vi "Symphony Operate.vi"() -> ()   [LabVIEW 2019]
uses:
  <userlib>/JY Symphony/NoiseCorr.ctl
  <userlib>/JY Symphony/AcqParState.ctl
  <userlib>/JY Symphony/SetAcqParMessage.ctl
panel:
  in  "Noise Corr":T1 caption="Noise Substraction"
  in  "SetArea":bool
  in  "Y Start":i32=255 min=1 max=255 step=1
  in  "X End":i32=1024 min=1 max=1024 step=1
  in  "Y End":i32=256 min=1 max=256 step=1
  in  "X Start":i32=1023 min=1 max=1023 step=1
  out "RemCom":bool
  in  "Server Running":bool
  out "TempReq":bool
  in  "Image mode":bool
  in  "T_Acq_Int":u32=1000 caption="T_Acq_Interval (ms)"
  out "T_AcqTime":u32
  out "Aquiring":bool
  out "Current Temp":dbl
  in  "ReadTemp":bool
  in  "Continuous Acq.":bool
  in  "AcquireImage":bool
  in  "Y Bins":i32=1 min=1 max=256 step=1
  out "ServerConn":refnum<k13>
  in  "Launch server":bool
  out "ClientConn":refnum<k13>
  out "Datas":i32[][][](array[numeric])
  out "Acq Time(ms)":u32
  in  "Accumulations":u16=1 min=1 step=1
  in  "Shutter Enable":bool=TRUE
  in  "Areas":i32[][](array[numeric])=[[1], [1], [1], [1024], [256], [1], [1]]
  in  "Int_time(ms)":u16=10 caption="Integration time(ms)"
  out "Initialized":bool
  in  "ADC":u16(ring) caption="Device Name" items=["ADC1:  20 kHz Tab 1", "ADC1:  50 kHz Tab 2"]
  in  "Gain":u16(ring) caption="Device Name" items=["Gain  0.6(x)"=10, "Gain  1.0(x)"=11, "Gain  2.0(x)"=12, "Gain  4.0(x)"=13, "Gain  6.7(x)"=8, "Gain 13.3(x)"=2]
  out "Name":string="ccd de test"
  out "FirmwareVersion":string="V1.89  CCD_3000"
  out "activeXPixels":i32=1024
  out "activeYPixels":i32=256
  in  "Uniques ID":u16(ring) items=["CCD100"]
  in  "Camera Name":u16(ring) items=["Symphony"]
  in  "Stop":bool
  out "error out":errorcluster
  in  "Init":bool
  in  "error in (no error)":errorcluster
  in  "Tab Control":enum32{"Spectre", "Image"}(tab)
  out "Delta":i32
  out "Max X Position":i32[](array[numeric])
  out "Spectral Graph":i32[][](graph)
  out "Max Intensity":i32[](array[numeric])
  out "Image Graph":i32[][](graph)
  # "Area#"
  # "X Origin"
  # "Y Origin"
  # "X Size"
  # "Y Size"
  # "X Bin"
  # "Y Bin"
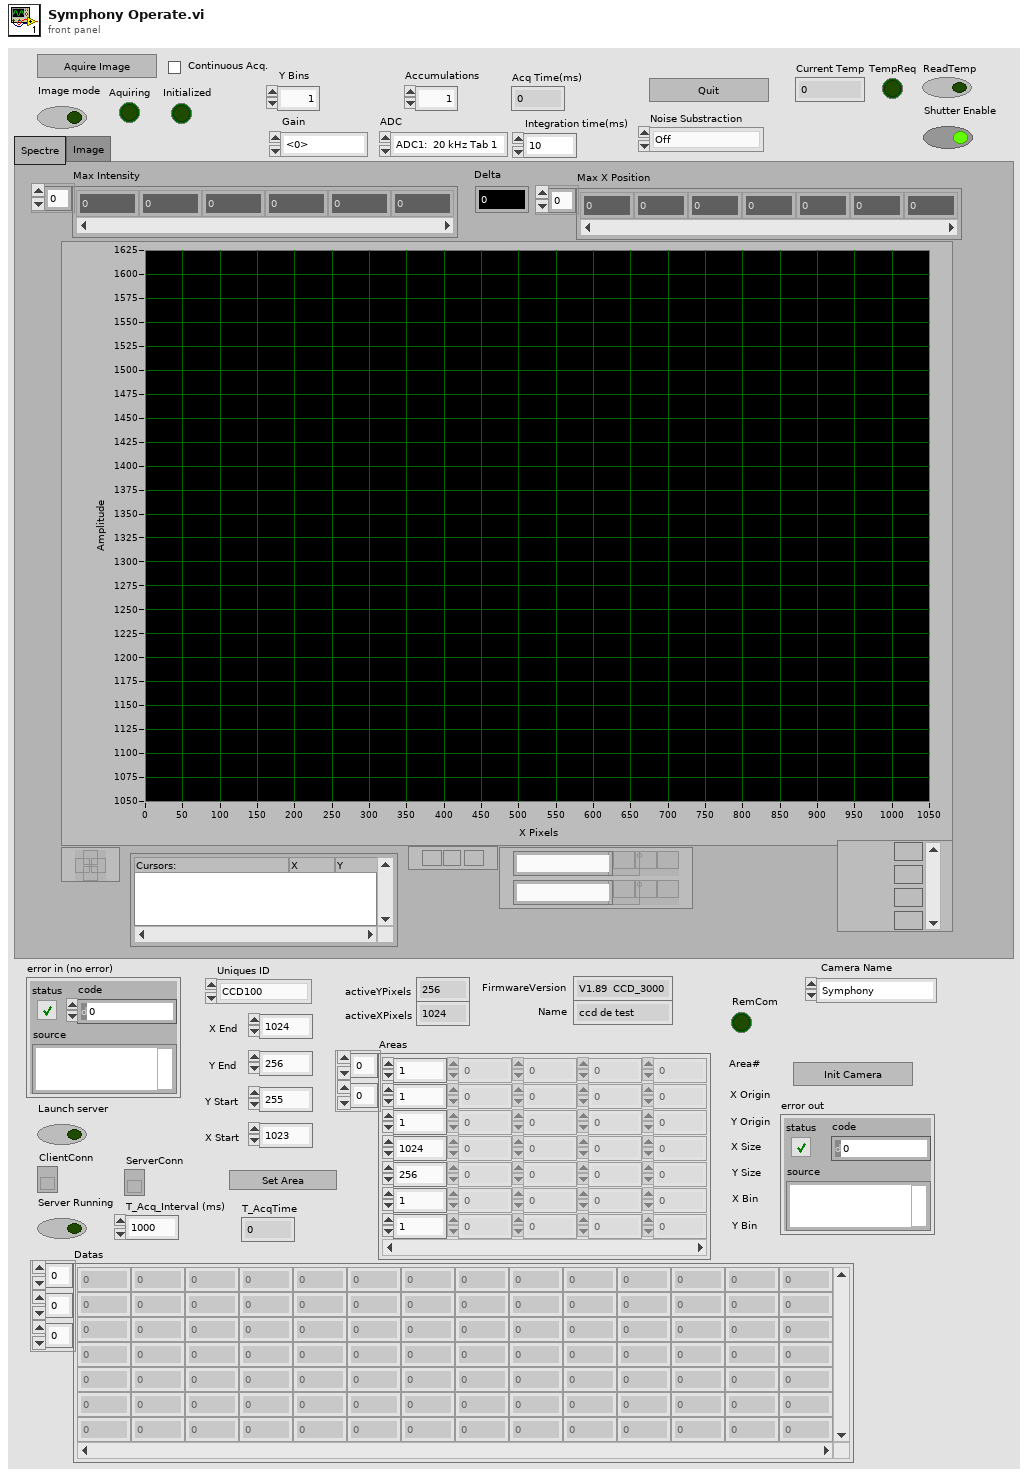
[diagram p1: front panel]
types:
  T1 = typedef "NoiseCorr.ctl" = enum16{"Off", "One For All Acq", "One For Every Acq"}
  T2 = cluster{"Message":string, "Data":variant, "Code":i32}
  T3 = enum16{"Read", "Write", "ReadWrite", "BufferedRead", "BufferedReadWrite"}
  T4 = typedef "AcqParState.ctl" = enum16{"All", "ADC", "Gain", "AcqType", "IntegTime", "Areas", "Error"}
  T5 = typedef "SetAcqParMessage.ctl" = cluster{"ADC":u16, "Gain":u16, "Int_time(ms)":u16, "Areas":i32[][], "Accumulation":u16}
  T6 = cluster{"Description":string, "GetNextADC":u16}[]
  T7 = typedef "LVStringsAndValuesArrayTypeDef_U16.ctl" = cluster{"String":string, "Value":u16}[]
  T8 = cluster{"StringsAndValues[]":T7, "Value":u16, "StringsAndValues[]":T7, "Value":u16, "Int_time(ms)":u16, "Areas":i32[][], "Current Temp":dbl, "Image mode":bool, "Shutter Enable":bool, "Accumulations":u16, u16}
  T9 = cluster{"Datas":i32[][][], "Current Temperature":dbl, "Image mode":bool}
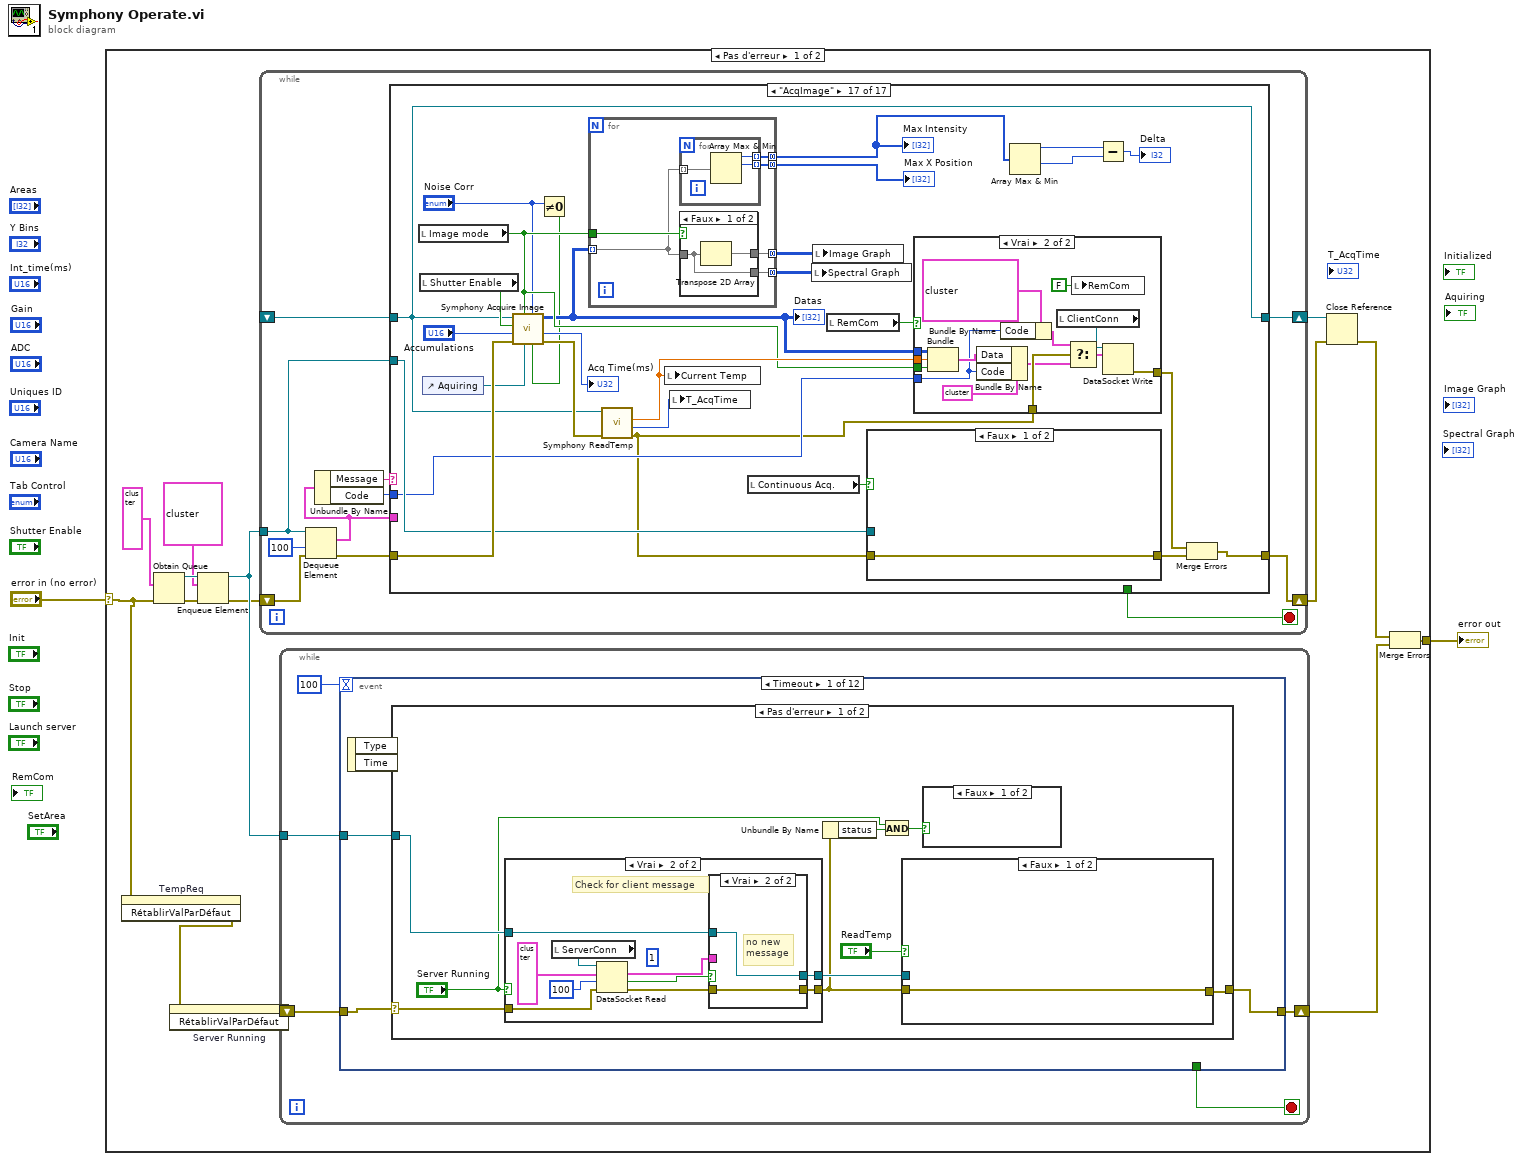
[diagram p0: block diagram]
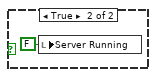
[diagram p2: hidden frame]
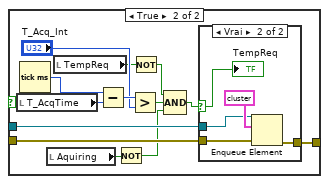
[diagram p3: hidden frame]
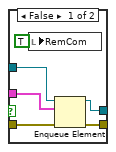
[diagram p6: hidden frame]
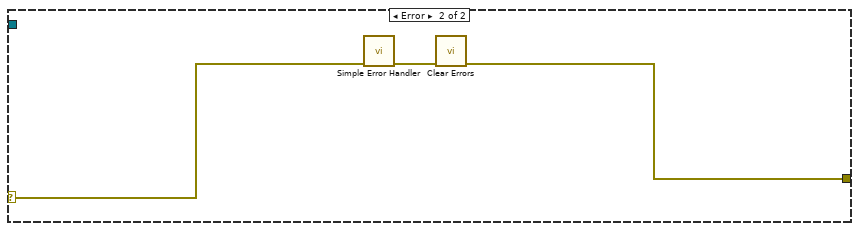
[diagram p7: hidden frame]
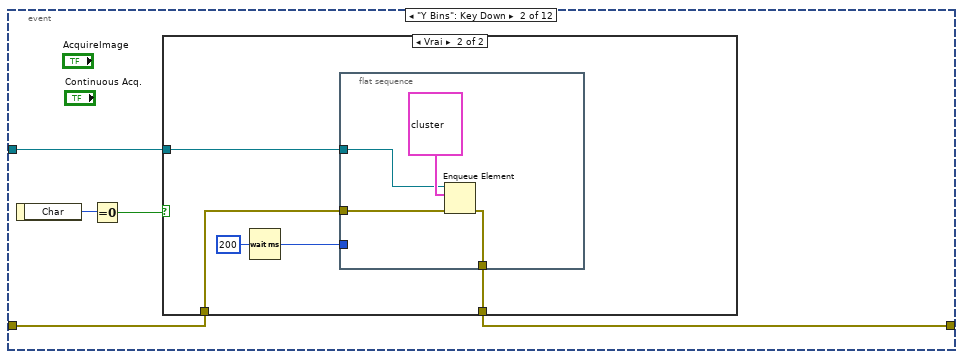
[diagram p8: hidden frame]
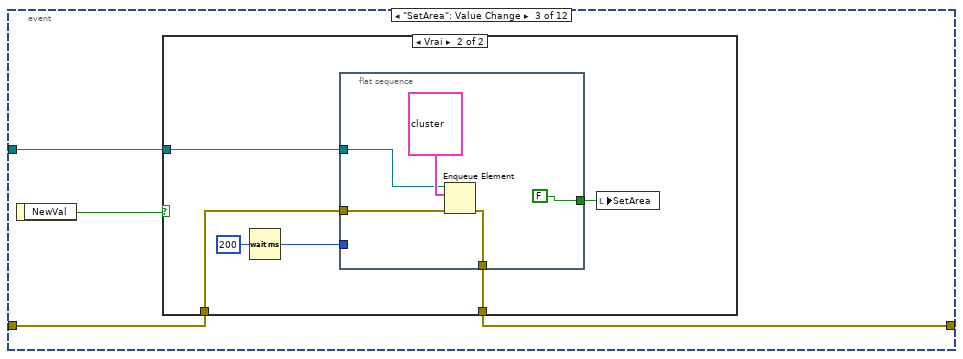
[diagram p10: hidden frame]
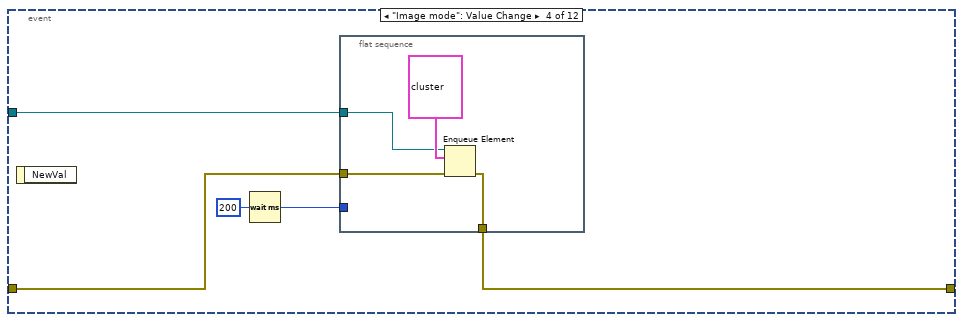
[diagram p12: hidden frame]
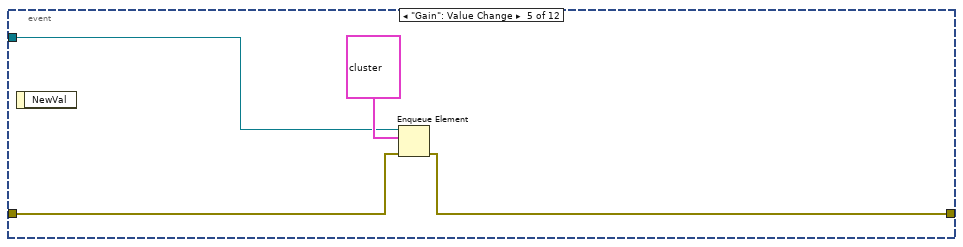
[diagram p13: hidden frame]
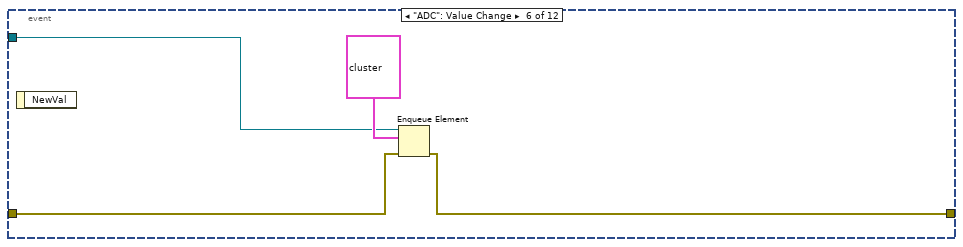
[diagram p14: hidden frame]
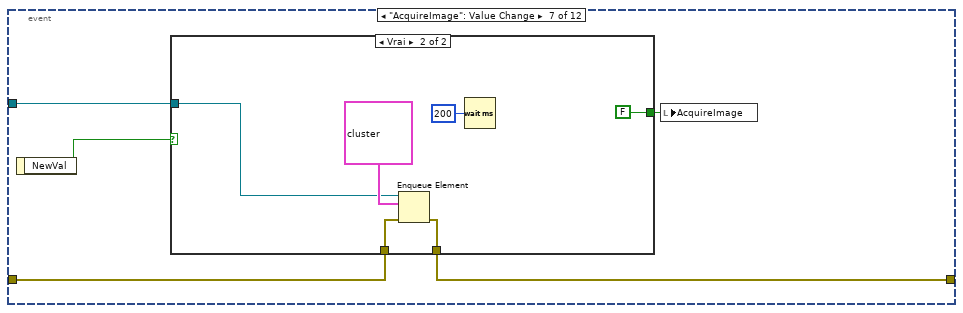
[diagram p15: hidden frame]
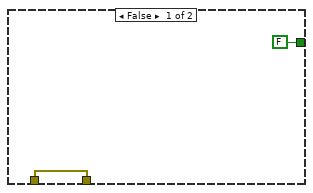
[diagram p16: hidden frame]
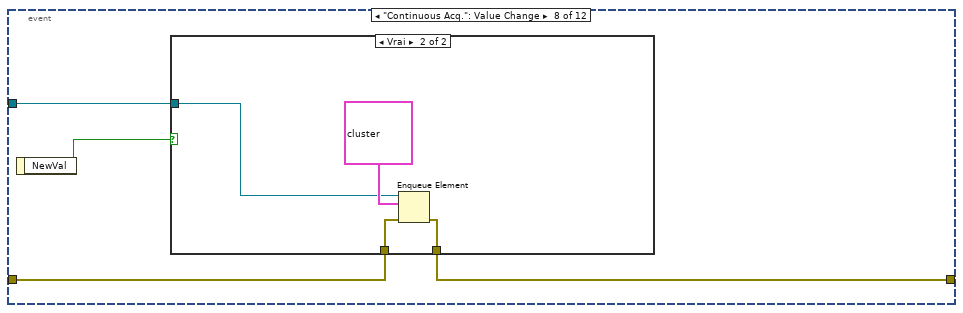
[diagram p17: hidden frame]
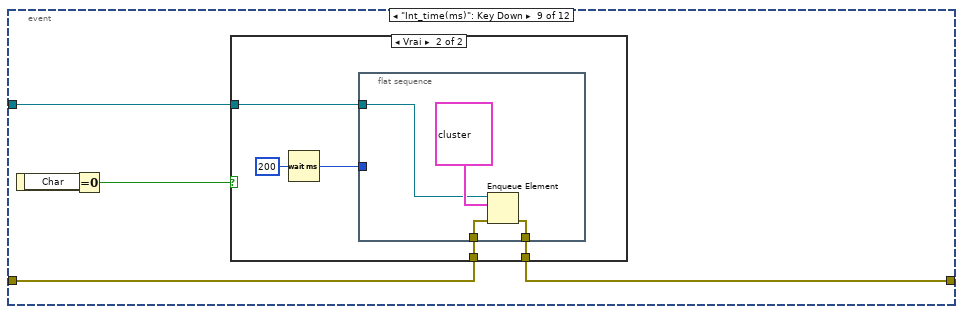
[diagram p19: hidden frame]
diagram:
  n1 = case shown="Pas d'erreur" "error in (no error)" {
    selector: "error in (no error)" -> [w4 w721]
    tunnel: [w14 w721] -> w1
    frame No Error {
      n2 = invoke on="TempReq" class="Bool (strict)" method="RétablirValParDéfaut"(error in=w4) -> (error out=w3:errorcluster)  [unwired: 2 in, 2 out]
      n3 = Obtain Queue(element data type=T2 {"Message"="", "Data"=variant, "Code"=0} ("element"), error in (no error)=w4) -> (queue out=w15:refnum<queue>, error out=w16:errorcluster)  [unwired: 3 in, 1 out]
      n4 = invoke on="Server Running" class="Bool (strict)" method="RétablirValParDéfaut"(error in=w3) -> (error out=w6:errorcluster)  [unwired: 2 in, 2 out]
      n5 = Enqueue Element(queue=w15, element=cluster{"Message":string, "Data":variant, i32} {"Message"="Init Prog", "Data"=variant, 0} ("ClassQueue"), error in (no error)=w16) -> (queue out=w13:refnum<queue>, error out=w5:errorcluster)  [unwired: 1 in, 1 out]
      n6 = while {
        shift-right: [w206] -> w8
        shift-left: w5 -> [w207]
        tunnel: w13 -> [w198]
        shift-right: [w202] -> w7
        shift-left: _ -> [w201]
        stop <- w203 stop-if-true
        n7 = Dequeue Element(queue=w198, timeout in ms (-1)=100, error in (no error)=w207) -> (element=w199:T2, error out=w205:errorcluster)  [unwired: 2 out]
        n8 = Unbundle By Name(w199) -> ("Message"=w204:string, "Code"=w197:i32)
        n9 = case shown="\"AcqImage\"" w204 {
          tunnel: [w208 w222 w245 w278 w319 w323 w351 w376 w423 w452 w487 w522 w556 w583 w608 w642 w664] -> w206
          tunnel: w205 -> [w209 w225 w232 w282 w314 w344 w350 w381 w428 w451 w486 w521 w555 w582 w611 w652 w682]
          tunnel: [TRUE FALSE FALSE _ _ _ _ _ _ _ _ _ _ _ _ _ _] -> w203
          tunnel: [w211 w223 w251 w292 w318 w321 w349 w375 w422 w453 w488 w523 w557 w584 w609 w641 w673] -> w202
          tunnel: w201 -> [w211 w223 w251 _ w313 w343 w349 w380 w427 w454 w489 w524 w558 w585 w610 w641 w673]
          tunnel: w199 -> [_ _ _ _ _ _ _ w378 w425 w450 w485 w520 w554 w581 _ w654 _]
          tunnel: w198 -> [_ _ w248 w276 _ _ _ _ _ _ _ _ _ _ _ w651 w676]
          tunnel: w197 -> [_ _ _ _ _ _ w348 w377 w424 w449 w484 w519 w553 w580 w606 _ w662]
          frame "Stop" {
            n10 = local read "Launch server"() -> (w210:bool)
            n11 = case shown="Vrai" w210 {
              tunnel: w209 -> [w213 w219]
              tunnel: [w213 w215] -> w208
              frame False {
              }
              frame True {
                n12 = local read "ServerConn"() -> (w218:refnum<k13>)
                n13 = local read "ClientConn"() -> (w220:refnum<k13>)
                n14 = DataSocket Close(8:w219, 11:w218) -> (0:w216:errorcluster)  [unwired: 1 in, 1 out]
                n15 = DataSocket Close(8:w219, 11:w220) -> (0:w217:errorcluster)  [unwired: 1 in, 1 out]
                n16 = local write "Server Running"(FALSE ("Server Running")) -> ()
                n17 = Merge Errors(w216, w217) -> (w215:errorcluster)
              }
            }
          }
          frame "Timeout", Default {
            n18 = call <vilib>:"General Error Handler.vi"("error in (no error)"=w225) -> ("error out"=w221:errorcluster)  [unwired: 10 in, 4 out]
            n19 = local write "error out"(w221) -> ()
            n20 = call <vilib>:"Clear Errors.vi"("error in (no error)"=w221) -> ("error out"=w222:errorcluster)  [unwired: 5 in, 1 out]
          }
          frame "Init Prog" {
            n21 = invoke on="Initialized" class="Bool (strict)" method="RétablirValParDéfaut"(error in=w232) -> (error out=w242:errorcluster)  [unwired: 2 in, 2 out]
            n22 = call <userlib>:"Symphony Read Det Uniq_ID.vi"("error in (no error)"=w232) -> ("error out"=w252:errorcluster, "Name"=w253:string[], "UniqueID"=w249:string[])  [unwired: 6 in, 2 out]
            n23 = call <userlib>:"Symphony GetProgPar.vi"("Param"=enum16{"InitVal", "Tous"}."InitVal", "error in"=w232) -> ("InitOnStart"=w233:bool, "Launch server"=w234:bool, "error out"=w229:errorcluster)  [unwired: 3 in, 8 out]
            n24 = Reverse 1D Array(array=u32[] [16711680, 16773120, 2359040, 131327, 3080307] ("Sous-tableau")) -> (reversed array=w243:u32[])
            n25 = property on="Camera Name" class="MDér (strict)"(error in=w252, "Strings []"=w253) -> (error out=w250:errorcluster)  [unwired: 1 in, 1 out]
            n26 = invoke on="Y Bins" class="DigNum (strict)" method="RétablirValParDéfaut"(error in=w242) -> (error out=w241:errorcluster)  [unwired: 2 in, 2 out]
            n27 = local write "Launch server"(w234) -> ()
            n28 = property on="Uniques ID" class="MDér (strict)"(error in=w250, "Strings []"=w249) -> (error out=w231:errorcluster)  [unwired: 1 in, 1 out]
            n29 = for {
              tunnel: cluster{dbl, u32}[] [{0.0, 0}, {10923.0, 0}, {21845.0, 0}, {32768.0, 0}, {43691.0, 0}, {54613.0, 0}] ("Z Scale.Marker Values[]") -> [w257] mode=indexing
              tunnel: w243 -> [w256] mode=indexing
              tunnel: [w255] -> w238 mode=indexing
              n30 = Bundle(cluster=w257, w256) -> (w255:cluster{dbl, u32})  [unwired: 1 in]
            }
            n31 = invoke on="Accumulations" class="DigNum (strict)" method="RétablirValParDéfaut"(error in=w241) -> (error out=w240:errorcluster)  [unwired: 2 in, 2 out]
            n32 = Merge Errors(w231, w229) -> (w230:errorcluster)
            n33 = invoke on="Areas" class="Arr (strict)" method="RétablirValParDéfaut"(error in=w240) -> (error out=w236:errorcluster)  [unwired: 2 in, 2 out]
            n34 = case shown="Vrai" w234 {
              tunnel: [w263 w266] -> w246
              tunnel: w230 -> [w263 w269]
              frame False {
              }
              frame True {
                n35 = DataSocket Open(8:w269, 10:T3."Write" ("mode"), 11:"dstp://localhost/SympClient" ("URL")) -> (0:w271:errorcluster, 3:→"ClientConn":refnum<k13>)  [unwired: 1 in]
                n36 = DataSocket Open(8:w271, 10:T3."Read" ("mode"), 11:"dstp://localhost/SympServer" ("URL")) -> (0:w266:errorcluster, 3:→"ServerConn":refnum<k13>)  [unwired: 1 in]
                n37 = Unbundle By Name(w266) -> ("status"=w265:bool)
                n38 = Not(x=w265) -> (.not. x?=w264:bool)
                n39 = local write "Server Running"(w264) -> ()
              }
            }
            n40 = property on="Image Graph" class="GraphInt (strict)"(error in=w232, "ZScale.MarkerVals[]"=w238) -> (error out=w239:errorcluster)  [unwired: 1 in, 1 out]
            n41 = invoke on="Image mode" class="Bool (strict)" method="RétablirValParDéfaut"(error in=w236) -> (error out=w235:errorcluster)  [unwired: 2 in, 2 out]
            n42 = case shown="Vrai" w233 {
              tunnel: w248 -> [_ w261]
              tunnel: w230 -> [w258 w260]
              tunnel: [w258 w259] -> w247
              frame False {
              }
              frame True {
                n43 = Enqueue Element(queue=w261, element=cluster{"Message":string, "Data":variant, i32} {"Message"="InitCam", "Data"=variant, 0} ("ClassQueue"), error in (no error)=w260) -> (error out=w259:errorcluster)  [unwired: 1 in, 2 out]
              }
            }
            n44 = invoke on="RemCom" class="Bool (strict)" method="RétablirValParDéfaut"(error in=w235) -> (error out=w227:errorcluster)  [unwired: 2 in, 2 out]
            n45 = invoke on="Noise Corr" class="Enum (strict)" method="RétablirValParDéfaut"(error in=w227) -> (error out=w226:errorcluster)  [unwired: 2 in, 2 out]
            n46 = Merge Errors(w226, w246, w247, w239) -> (w245:errorcluster)
          }
          frame "InitCam" {
            n47 = call <vilib>:"Set Busy.vi"("error in (no error)"=w282) -> ("error out"=w281:errorcluster)  [unwired: 9 in, 1 out]
            n48 = local read "Camera Name"() -> (w300:u16)
            n49 = property on="Uniques ID" class="MDér (strict)"(error in=w281) -> (error out=w297:errorcluster, "Strings []"=w301:string[])  [unwired: 1 in, 1 out]
            n50 = To Long Integer(number=w300) -> (32bit integer=w299:i32)
            n51 = Index Array(array=w301, index=w299) -> (element=w298:string)
            n52 = call <userlib>:"Symphony Init.vi"("error In"=w297, "Unique id:"=w298) -> ("error out"=w293:errorcluster, "activeYPixels"=→"activeYPixels":i32, "activeXPixels"=→"activeXPixels":i32, "JYCCDLib.IJYCCDReqd"=w294:refnum<k7>, "Name"=→"Name":string, "FirmwareVersion"=→"FirmwareVersion":string)  [unwired: 3 in]
            n53 = call <userlib>:"Symphony Init ADC & Gain.vi"("error in (no error)"=w293, "JYCCDLib.IJYCCDReqd"=w294) -> ("error out"=w291:errorcluster, "ADC Values"=w289:T6, "Gain Values"=w284:T6, "JYCCDLib.IJYCCDReqd Out"=w292:refnum<k7>, "CurrentADC"=w287:i32, "CurrentGain"=w285:i32)  [unwired: 4 in]
            n54 = To Unsigned Word Integer(number=w285) -> (unsigned 16bit integer=w286:u16)
            n55 = To Unsigned Word Integer(number=w287) -> (unsigned 16bit integer=w283:u16)
            n56 = property on="ADC" class="MDér (strict)"(error in=w291, "StringsAndValues[]"=w289, "Value"=w283) -> (error out=w288:errorcluster)  [unwired: 1 in, 1 out]
            n57 = property on="Gain" class="MDér (strict)"(error in=w291, "StringsAndValues[]"=w284, "Value"=w286) -> (error out=w290:errorcluster)  [unwired: 1 in, 1 out]
            n58 = Merge Errors(w290, w288) -> (w277:errorcluster)
            n59 = case shown="Pas d'erreur" w277 {
              selector: w277 -> [w306 w308]
              tunnel: w276 -> [w305 _]
              tunnel: [w304 w308] -> w275
              frame No Error {
                n60 = Enqueue Element(queue=w305, element=T2 {"Message"="InitSetupAll", "Data"=variant, "Code"=1}, error in (no error)=w306) -> (error out=w304:errorcluster)  [unwired: 1 in, 2 out]
              }
              frame Error {
              }
            }
            n61 = call <vilib>:"Clear Errors.vi"("error in (no error)"=w277) -> ("error out"=w280:errorcluster)  [unwired: 5 in, 1 out]
            n62 = call <vilib>:"Unset Busy.vi"("error in (no error)"=w280) -> ("error out"=w279:errorcluster)  [unwired: 10 in]
            n63 = Merge Errors(w275, w279) -> (w278:errorcluster)
          }
          frame "AcqSetupAll" {
            (unwired) 0 ("Code")
            n64 = local read "Int_time(ms)"() -> (w312:u16)
            n65 = local read "Areas"() -> (w309:i32[][])
            n66 = local read "ADC"() -> (w311:u16)
            n67 = local read "Gain"() -> (w310:u16)
            n68 = To Long Integer(number=w311) -> (32bit integer=w316:i32)
            n69 = To Long Integer(number=w310) -> (32bit integer=w317:i32)
            n70 = call <userlib>:"Symphony Setup V2.vi"("areas :"=w309, "Function"=AcqParState."All", "Int_time(ms)"=w312, "error in (no error)"=w314, "Gain"=w317, "Select ADC"=w316, "JYCCDLib.IJYCCDReqd"=w313) -> ("error out"=w319:errorcluster, "JYCCDLib.IJYCCDReqdOut"=w318:refnum<k7>)  [unwired: 2 in, 1 out]
          }
          frame "InitSetupAll" {
            w326 = u16 0 items=["° Celsius", "Kelvin", "° Farenheit"] ("units")
            w338 = 256 ("Y Start")
            w340 = 1 ("Y Start")
            n71 = call <userlib>:"Symphony GetProgPar.vi"("Param"=enum16{"InitVal", "Tous"}."Tous", "error in"=w344) -> ("Y Bins"=w335:i32, "X Start"=w337:i32, "X End"=w339:i32, "ImageMode"=w336:bool, "Shutter Enable"=w330:bool, "ADC"=w332:u16, "Gain"=w333:u16, "Int_time(ms)"=w329:i16, "error out"=w342:errorcluster)  [unwired: 3 in, 2 out]
            n72 = local write "Shutter Enable"(w330) -> ()
            n73 = local write "Int_time(ms)"(w329) -> ()
            n74 = local write "Gain"(w333) -> ()
            n75 = local write "ADC"(w332) -> ()
            n76 = local write "Image mode"(w336) -> ()
            n77 = local write "Y Bins"(w335) -> ()
            n78 = local write "X Start"(w337) -> ()
            n79 = local write "X End"(w339) -> ()
            n80 = call <userlib>:"Symphony Format Area.vi"("Y Start"=w340, "Y End"=w338, "ImageMode"=w336, "error in (no error)"=w342, "X Start"=w337, "X End"=w339, "numAreas"=w335) -> ("error out"=w341:errorcluster, "areas :"=w334:i32[][])  [unwired: 1 in, 1 out]
            n81 = local write "Y End"(w338) -> ()
            n82 = local write "Areas"(w334) -> ()
            n83 = local write "Y Start"(w340) -> ()
            n84 = To Long Integer(number=w332) -> (32bit integer=w346:i32)
            n85 = To Long Integer(number=w333) -> (32bit integer=w347:i32)
            n86 = call <userlib>:"Symphony Setup V2.vi"("areas :"=w334, "Function"=AcqParState."All", "Int_time(ms)"=w329, "error in (no error)"=w341, "Gain"=w347, "Select ADC"=w346, "JYCCDLib.IJYCCDReqd"=w343) -> ("error out"=w324:errorcluster, "JYCCDLib.IJYCCDReqdOut"=w322:refnum<k7>)  [unwired: 2 in, 1 out]
            n87 = call <userlib>:"Symphony ReadTemp.vi"("error in (no error)"=w324, "units"=w326, "JYCCDLib.IJYCCDReqd"=w322) -> ("error out"=w323:errorcluster, "AcqTime"=w325:u32, "Current Temperature"=w327:dbl, "reference out"=w321:refnum<k7>)  [unwired: 4 in]
            n88 = local write "T_AcqTime"(w325) -> ()
            n89 = local write "Current Temp"(w327) -> ()
            n90 = Unbundle By Name(w323) -> ("status"=w328:bool)
            n91 = Not(x=w328) -> (.not. x?=w320:bool)
            n92 = local write "Initialized"(w320) -> ()
          }
          frame "CheckStatus" {
            n93 = local read "RemCom"() -> (w352:bool)
            n94 = case shown="Vrai" w352 {
              selector: w352 -> [_ w360]
              tunnel: w350 -> [w353 w371]
              tunnel: [w353 w370] -> w351
              tunnel: w348 -> [_ w362]
              frame False {
              }
              frame True {
                n95 = Not(x=w360) -> (.not. x?=w359:bool)
                n96 = property on="ADC" class="MDér (strict)"() -> ("StringsAndValues[]"=w369:T7, "Value"=w368:u16)  [unwired: 2 in, 2 out]
                n97 = property on="Gain" class="MDér (strict)"() -> ("StringsAndValues[]"=w367:T7, "Value"=w366:u16)  [unwired: 2 in, 2 out]
                n98 = local write "RemCom"(w359) -> ()
                n99 = local read "Accumulations"() -> (w356:u16)
                n100 = local read "Image mode"() -> (w358:bool)
                n101 = local read "Int_time(ms)"() -> (w364:u16)
                n102 = local read "Current Temp"() -> (w361:dbl)
                n103 = local read "Shutter Enable"() -> (w357:bool)
                n104 = local read "Noise Corr"() -> (w355:T1)
                n105 = local read "Areas"() -> (w363:i32[][])
                n106 = To Unsigned Word Integer(number=w355) -> (unsigned 16bit integer=w354:u16)
                n107 = Bundle("StringsAndValues[]"=w369, "Value"=w368, "StringsAndValues[]"=w367, "Value"=w366, "Int_time(ms)"=w364, "Areas"=w363, "Current Temp"=w361, "Image mode"=w358, "Shutter Enable"=w357, "Accumulations"=w356, w354) -> (w365:T8)  [unwired: 1 in]
                n108 = local read "ClientConn"() -> (w374:refnum<k13>)
                n109 = Bundle By Name(cluster=T2 {"Message"="Status", "Data"=variant, "Code"=0} ("ClassQueue"), "Data"=w365, "Code"=w362) -> (w372:T2)
                n110 = DataSocket Write(8:w371, 10:w372, 11:w374) -> (0:w370:errorcluster)  [unwired: 1 in, 2 out]
              }
            }
          }
          frame "SetArea" {
            n111 = local read "RemCom"() -> (w379:bool)
            n112 = case shown="Faux" w379 {
              selector: w379 -> [_ w420]
              tunnel: w381 -> [w394 w411]
              tunnel: w380 -> [w393 w416]
              tunnel: [w392 w415] -> w375
              tunnel: w378 -> [_ w413]
              tunnel: w377 -> [_ w409]
              tunnel: [w384 w405] -> w376
              frame False {
                n113 = local read "Y Bins"() -> (w388:i32)
                n114 = call <userlib>:"Symphony Format Area.vi"("Y Start"="Y Start", "Y End"="Y End", "ImageMode"="Image mode", "error in (no error)"=w394, "X Start"="X Start", "X End"="X End", "numAreas"=w388) -> ("error out"=w390:errorcluster, "areas :"=w389:i32[][])  [unwired: 1 in, 1 out]
                n115 = local write "Areas"(w389) -> ()
                n116 = call <userlib>:"Symphony Setup V2.vi"("areas :"=w389, "Function"=AcqParState."Areas", "error in (no error)"=w390, "JYCCDLib.IJYCCDReqd"=w393) -> ("error out"=w384:errorcluster, "JYCCDLib.IJYCCDReqdOut"=w392:refnum<k7>)  [unwired: 5 in, 1 out]
              }
              frame True {
                w407 = T2 {"Message"="CommandError", "Data"=variant, "Code"=0} ("ClassQueue")
                n117 = Not(x=w420) -> (.not. x?=w421:bool)
                n118 = local write "RemCom"(w421) -> ()
                n119 = Unbundle By Name(w413) -> ("Data"=w412:variant)
                n120 = Bundle("Areas"=i32[][] [[1], [1], [1], [1024], [256], [1], [1]], TRUE) -> (w400:cluster{"Areas":i32[][], bool})  [unwired: 1 in]
                n121 = Variant To Data(error in=w411, type=w400, Variant=w412) -> (data=w414:cluster{"Areas":i32[][], bool}, error out=w410:errorcluster)
                n122 = Unbundle(w414) -> ("Areas"=w398:i32[][], w399:bool)
                n123 = Bundle By Name(cluster=w407, "Code"=w409) -> ()  [unwired: 1 out]
                n124 = call <userlib>:"Symphony Setup V2.vi"("areas :"=w398, "Function"=AcqParState."Areas", "error in (no error)"=w410, "JYCCDLib.IJYCCDReqd"=w416) -> ("error out"=w403:errorcluster, "JYCCDLib.IJYCCDReqdOut"=w415:refnum<k7>)  [unwired: 5 in, 1 out]
                n125 = local write "Image mode"(w399) -> ()
                n126 = local write "Areas"(w398) -> ()
                n127 = Array Size(array=w398) -> (size(s)=w397:i32[])
                n128 = Bundle By Name(cluster=T2 {"Message"="Area", "Data"=variant, "Code"=0} ("ClassQueue"), "Code"=w409) -> (w408:T2)
                n129 = Select(t=w407, s=w403, f=w408) -> (s? t:f=w406:T2)
                n130 = local read "ClientConn"() -> (w418:refnum<k13>)
                n131 = Index Array(array=w397, index=1) -> (element=w395:i32)
                n132 = DataSocket Write(10:w406, 11:w418) -> (0:w404:errorcluster)  [unwired: 2 in, 2 out]
                n133 = local write "Y Bins"(w395) -> ()
                n134 = Merge Errors(w404, w403) -> (w405:errorcluster)
              }
            }
          }
          frame "SetShutterEn" {
            n135 = local read "RemCom"() -> (w426:bool)
            n136 = case shown="Vrai" w426 {
              selector: w426 -> [_ w446]
              tunnel: w428 -> [w429 w441]
              tunnel: w427 -> [w430 w433]
              tunnel: [w430 w433] -> w422
              tunnel: w425 -> [_ w443]
              tunnel: w424 -> [_ w440]
              tunnel: [w429 w436] -> w423
              frame False {
              }
              frame True {
                w438 = T2 {"Message"="CommandError", "Data"=variant, "Code"=0} ("ClassQueue")
                n137 = Not(x=w446) -> (.not. x?=w447:bool)
                n138 = local write "RemCom"(w447) -> ()
                n139 = Unbundle By Name(w443) -> ("Data"=w442:variant)
                n140 = Variant To Data(error in=w441, type=TRUE, Variant=w442) -> (data=w431:bool, error out=w434:errorcluster)
                n141 = local write "Shutter Enable"(w431) -> ()
                n142 = Bundle By Name(cluster=w438, "Code"=w440) -> ()  [unwired: 1 out]
                n143 = Bundle By Name(cluster=T2 {"Message"="ShutterEn", "Data"=variant, "Code"=0} ("ClassQueue"), "Code"=w440, "Data"=w431) -> (w439:T2)
                n144 = Select(t=w438, s=w434, f=w439) -> (s? t:f=w437:T2)
                n145 = local read "ClientConn"() -> (w444:refnum<k13>)
                n146 = DataSocket Write(10:w437, 11:w444) -> (0:w435:errorcluster)  [unwired: 2 in, 2 out]
                n147 = Merge Errors(w435, w434) -> (w436:errorcluster)
              }
            }
          }
          frame "SetGain" {
            n148 = local read "RemCom"() -> (w448:bool)
            n149 = case shown="Vrai" w448 {
              selector: w448 -> [_ w462]
              tunnel: w454 -> [w461 w482]
              tunnel: [w460 w481] -> w453
              tunnel: [w458 w470] -> w452
              tunnel: w451 -> [w457 w468]
              tunnel: w450 -> [_ w480]
              tunnel: w449 -> [_ w466]
              frame False {
                n150 = local read "Gain"() -> (w456:u16)
                n151 = To Long Integer(number=w456) -> (32bit integer=w455:i32)
                n152 = call <userlib>:"Symphony Setup V2.vi"("Function"=AcqParState."Gain", "error in (no error)"=w457, "Gain"=w455, "JYCCDLib.IJYCCDReqd"=w461) -> ("error out"=w458:errorcluster, "JYCCDLib.IJYCCDReqdOut"=w460:refnum<k7>)  [unwired: 5 in, 1 out]
              }
              frame True {
                n153 = Not(x=w462) -> (.not. x?=w463:bool)
                n154 = Unbundle By Name(w480) -> ("Data"=w473:variant)
                n155 = local write "RemCom"(w463) -> ()
                n156 = Variant To Data(error in=w468, type=0 ("Gain"), Variant=w473) -> (data=w464:i32, error out=w471:errorcluster)
                n157 = call <userlib>:"Symphony Setup V2.vi"("Function"=AcqParState."Gain", "error in (no error)"=w471, "Gain"=w464, "JYCCDLib.IJYCCDReqd"=w482) -> ("error out"=w469:errorcluster, "JYCCDLib.IJYCCDReqdOut"=w481:refnum<k7>)  [unwired: 5 in, 1 out]
                n158 = Bundle By Name(cluster=T2 {"Message"="Gain", "Data"=variant, "Code"=0} ("ClassQueue"), "Data"=w464, "Code"=w466) -> (w476:T2)
                n159 = local write "Gain"(w464) -> ()
                n160 = Bundle By Name(cluster=T2 {"Message"="CommandError", "Data"=variant, "Code"=0} ("ClassQueue"), "Code"=w466) -> (w465:T2)
                n161 = Select(t=w465, s=w469, f=w476) -> (s? t:f=w477:T2)
                n162 = local read "ClientConn"() -> (w478:refnum<k13>)
                n163 = DataSocket Write(10:w477, 11:w478) -> (0:w474:errorcluster)  [unwired: 2 in, 2 out]
                n164 = Merge Errors(w474, w469) -> (w470:errorcluster)
              }
            }
          }
          frame "SetADC" {
            n165 = local read "RemCom"() -> (w483:bool)
            n166 = case shown="Vrai" w483 {
              selector: w483 -> [_ w497]
              tunnel: w489 -> [w496 w517]
              tunnel: [w495 w516] -> w488
              tunnel: [w493 w505] -> w487
              tunnel: w486 -> [w492 w503]
              tunnel: w485 -> [_ w515]
              tunnel: w484 -> [_ w501]
              frame False {
                n167 = local read "ADC"() -> (w491:u16)
                n168 = To Long Integer(number=w491) -> (32bit integer=w490:i32)
                n169 = call <userlib>:"Symphony Setup V2.vi"("Function"=AcqParState."ADC", "error in (no error)"=w492, "Gain"=w490, "JYCCDLib.IJYCCDReqd"=w496) -> ("error out"=w493:errorcluster, "JYCCDLib.IJYCCDReqdOut"=w495:refnum<k7>)  [unwired: 5 in, 1 out]
              }
              frame True {
                n170 = Unbundle By Name(w515) -> ("Data"=w508:variant)
                n171 = Not(x=w497) -> (.not. x?=w498:bool)
                n172 = local write "RemCom"(w498) -> ()
                n173 = Variant To Data(error in=w503, type=0 ("Gain"), Variant=w508) -> (data=w499:i32, error out=w506:errorcluster)
                n174 = call <userlib>:"Symphony Setup V2.vi"("Function"=AcqParState."ADC", "error in (no error)"=w506, "Gain"=w499, "JYCCDLib.IJYCCDReqd"=w517) -> ("error out"=w504:errorcluster, "JYCCDLib.IJYCCDReqdOut"=w516:refnum<k7>)  [unwired: 5 in, 1 out]
                n175 = Bundle By Name(cluster=T2 {"Message"="ADC", "Data"=variant, "Code"=0} ("ClassQueue"), "Data"=w499, "Code"=w501) -> (w511:T2)
                n176 = local write "ADC"(w499) -> ()
                n177 = Bundle By Name(cluster=T2 {"Message"="CommandError", "Data"=variant, "Code"=0} ("ClassQueue"), "Code"=w501) -> (w500:T2)
                n178 = local read "ClientConn"() -> (w513:refnum<k13>)
                n179 = Select(t=w500, s=w504, f=w511) -> (s? t:f=w512:T2)
                n180 = DataSocket Write(10:w512, 11:w513) -> (0:w509:errorcluster)  [unwired: 2 in, 2 out]
                n181 = Merge Errors(w509, w504) -> (w505:errorcluster)
              }
            }
          }
          frame "SetInteg" {
            n182 = local read "RemCom"() -> (w518:bool)
            n183 = case shown="Vrai" w518 {
              selector: w518 -> [_ w531]
              tunnel: w524 -> [w530 w547]
              tunnel: [w529 w546] -> w523
              tunnel: [w527 w540] -> w522
              tunnel: w521 -> [w526 w538]
              tunnel: w520 -> [_ w551]
              tunnel: w519 -> [_ w533]
              frame False {
                n184 = local read "Int_time(ms)"() -> (w525:u16)
                n185 = call <userlib>:"Symphony Setup V2.vi"("Function"=AcqParState."IntegTime", "Int_time(ms)"=w525, "error in (no error)"=w526, "JYCCDLib.IJYCCDReqd"=w530) -> ("error out"=w527:errorcluster, "JYCCDLib.IJYCCDReqdOut"=w529:refnum<k7>)  [unwired: 5 in, 1 out]
              }
              frame True {
                n186 = Not(x=w531) -> (.not. x?=w532:bool)
                n187 = Unbundle By Name(w551) -> ("Data"=w550:variant)
                n188 = local write "RemCom"(w532) -> ()
                n189 = Variant To Data(error in=w538, type=u16 10 ("Int_time(ms)"), Variant=w550) -> (data=w536:u16, error out=w537:errorcluster)
                n190 = call <userlib>:"Symphony Setup V2.vi"("Function"=AcqParState."IntegTime", "Int_time(ms)"=w536, "error in (no error)"=w537, "JYCCDLib.IJYCCDReqd"=w547) -> ("error out"=w541:errorcluster, "JYCCDLib.IJYCCDReqdOut"=w546:refnum<k7>)  [unwired: 5 in, 1 out]
                n191 = Bundle By Name(cluster=T2 {"Message"="Integration", "Data"=variant, "Code"=0} ("ClassQueue"), "Data"=w536, "Code"=w533) -> (w542:T2)
                n192 = Bundle By Name(cluster=T2 {"Message"="CommandError", "Data"=variant, "Code"=0} ("ClassQueue"), "Code"=w533) -> (w534:T2)
                n193 = local read "ClientConn"() -> (w544:refnum<k13>)
                n194 = local write "Int_time(ms)"(w536) -> ()
                n195 = Select(t=w534, s=w541, f=w542) -> (s? t:f=w543:T2)
                n196 = DataSocket Write(10:w543, 11:w544) -> (0:w539:errorcluster)  [unwired: 2 in, 2 out]
                n197 = Merge Errors(w539, w541) -> (w540:errorcluster)
              }
            }
          }
          frame "SetAcc" {
            n198 = local read "RemCom"() -> (w552:bool)
            n199 = case shown="Vrai" w552 {
              selector: w552 -> [_ w564]
              tunnel: w558 -> [w560 w561]
              tunnel: [w560 w561] -> w557
              tunnel: [w559 w571] -> w556
              tunnel: w555 -> [w559 w569]
              tunnel: w554 -> [_ w578]
              tunnel: w553 -> [_ w566]
              frame False {
              }
              frame True {
                n200 = Not(x=w564) -> (.not. x?=w565:bool)
                n201 = Unbundle By Name(w578) -> ("Data"=w577:variant)
                n202 = local write "RemCom"(w565) -> ()
                n203 = Variant To Data(error in=w569, type=u16 10 ("Int_time(ms)"), Variant=w577) -> (data=w563:u16, error out=w562:errorcluster)
                n204 = Bundle By Name(cluster=T2 {"Message"="Accumulation", "Data"=variant, "Code"=0} ("ClassQueue"), "Data"=w563, "Code"=w566) -> (w572:T2)
                n205 = Bundle By Name(cluster=T2 {"Message"="CommandError", "Data"=variant, "Code"=0} ("ClassQueue"), "Code"=w566) -> (w567:T2)
                n206 = local write "Accumulations"(w563) -> ()
                n207 = local read "ClientConn"() -> (w574:refnum<k13>)
                n208 = Select(t=w567, s=w562, f=w572) -> (s? t:f=w573:T2)
                n209 = DataSocket Write(10:w573, 11:w574) -> (0:w570:errorcluster)  [unwired: 2 in, 2 out]
                n210 = Merge Errors(w570, w562) -> (w571:errorcluster)
              }
            }
          }
          frame "SetNoiseMode" {
            n211 = local read "RemCom"() -> (w579:bool)
            n212 = case shown="Vrai" w579 {
              selector: w579 -> [_ w591]
              tunnel: w585 -> [w587 w588]
              tunnel: [w587 w588] -> w584
              tunnel: [w586 w598] -> w583
              tunnel: w582 -> [w586 w596]
              tunnel: w581 -> [_ w605]
              tunnel: w580 -> [_ w593]
              frame False {
              }
              frame True {
                n213 = Not(x=w591) -> (.not. x?=w592:bool)
                n214 = Unbundle By Name(w605) -> ("Data"=w604:variant)
                n215 = local write "RemCom"(w592) -> ()
                n216 = Variant To Data(error in=w596, type=u16 10 ("Int_time(ms)"), Variant=w604) -> (data=w590:u16, error out=w589:errorcluster)
                n217 = Bundle By Name(cluster=T2 {"Message"="NoiseMode", "Data"=variant, "Code"=0} ("ClassQueue"), "Data"=w590, "Code"=w593) -> (w599:T2)
                n218 = Bundle By Name(cluster=T2 {"Message"="CommandError", "Data"=variant, "Code"=0} ("ClassQueue"), "Code"=w593) -> (w594:T2)
                n219 = local read "ClientConn"() -> (w601:refnum<k13>)
                n220 = local write "Noise Corr"(w590) -> ()
                n221 = Select(t=w594, s=w589, f=w599) -> (s? t:f=w600:T2)
                n222 = DataSocket Write(10:w600, 11:w601) -> (0:w597:errorcluster)  [unwired: 2 in, 2 out]
                n223 = Merge Errors(w597, w589) -> (w598:errorcluster)
              }
            }
          }
          frame "AcqTemp" {
            n224 = local read "RemCom"() -> (w607:bool)
            n225 = case shown="Vrai" w607 {
              selector: w607 -> [_ w634]
              tunnel: w611 -> [w619 w639]
              tunnel: w610 -> [w618 w638]
              tunnel: [w617 w622] -> w609
              tunnel: [w613 w623] -> w608
              tunnel: w606 -> [_ w624]
              frame False {
                w616 = u16 0 items=["° Celsius", "Kelvin", "° Farenheit"] ("units")
                n226 = call <userlib>:"Symphony ReadTemp.vi"("error in (no error)"=w619, "units"=w616, "JYCCDLib.IJYCCDReqd"=w618) -> ("error out"=w614:errorcluster, "AcqTime"=w615:u32, "Current Temperature"=w612:dbl, "reference out"=w617:refnum<k7>)  [unwired: 4 in]
                n227 = local write "T_AcqTime"(w615) -> ()
                n228 = flat-sequence {
                  tunnel: w614 -> [w620]
                  tunnel: [w620] -> w613
                  frame #0 {
                    n229 = local write "TempReq"(FALSE) -> ()
                  }
                }
                n230 = local write "Current Temp"(w612) -> ()
              }
              frame True {
                w637 = u16 0 items=["° Celsius", "Kelvin", "° Farenheit"] ("units")
                n231 = Not(x=w634) -> (.not. x?=w635:bool)
                n232 = local write "RemCom"(w635) -> ()
                n233 = call <userlib>:"Symphony ReadTemp.vi"("error in (no error)"=w639, "units"=w637, "JYCCDLib.IJYCCDReqd"=w638) -> ("error out"=w625:errorcluster, "AcqTime"=w636:u32, "Current Temperature"=w626:dbl, "reference out"=w622:refnum<k7>)  [unwired: 4 in]
                "Current Temp" <- w626
                n234 = local write "T_AcqTime"(w636) -> ()
                n235 = Bundle By Name(cluster=T2 {"Message"="Integration", "Data"=variant, "Code"=0} ("ClassQueue"), "Data"=w626, "Code"=w624) -> (w630:T2)
                n236 = Bundle By Name(cluster=T2 {"Message"="CommandError", "Data"=variant, "Code"=0} ("ClassQueue"), "Code"=w624) -> (w627:T2)
                n237 = local read "ClientConn"() -> (w632:refnum<k13>)
                n238 = Select(t=w627, s=w625, f=w630) -> (s? t:f=w631:T2)
                n239 = DataSocket Write(10:w631, 11:w632) -> (0:w629:errorcluster)  [unwired: 2 in, 2 out]
                n240 = Merge Errors(w629, w625) -> (w623:errorcluster)
              }
            }
          }
          frame "SetAcqPar" {
            n241 = Unbundle By Name(w654) -> ("Data"=w653:variant)
            n242 = Variant To Data(error in=w652, type=T5 {"ADC"=0, "Gain"=0, "Int_time(ms)"=10, "Areas"=[[1], [1], [1], [1024], [256], [1], [1]], "Accumulation"=0}, Variant=w653) -> (data=w647:T5, error out=w649:errorcluster)
            n243 = Unbundle By Name(w647) -> ("ADC"=w646:u16, "Gain"=w645:u16, "Int_time(ms)"=w644:u16, "Areas"=w643:i32[][], "Accumulation"=w640:u16)
            n244 = local write "Accumulations"(w640) -> ()
            n245 = local write "Int_time(ms)"(w644) -> ()
            n246 = local write "Areas"(w643) -> ()
            n247 = local write "ADC"(w646) -> ()
            n248 = local write "Gain"(w645) -> ()
            n249 = Enqueue Element(queue=w651, element=T2 {"Message"="AcqSetupAll", "Data"=variant, "Code"=0}, error in (no error)=w649) -> (error out=w642:errorcluster)  [unwired: 1 in, 2 out]
          }
          frame "AcqImage" {
            n250 = local read "Image mode"() -> (w659:bool)
            n251 = local read "Shutter Enable"() -> (w681:bool)
            n252 = control-ref of="Aquiring"() -> (w675:refnum<vi>)
            n253 = Not Equal To 0?(x="Noise Corr") -> (x != 0?=w655:bool)
            n254 = call <userlib>:"Symphony Acquire Image.vi"("Noise Substract"=w655, "Noise Mode"="Noise Corr", "AcqBusy"=w675, "ImageMode"=w659, "error in"=w682, "Accumulations"="Accumulations", "ShutterEnable"=w681, "JYCCDLib.IJYCCDReqd"=w673) -> ("error out"=w674:errorcluster, "Acq Time(ms)"=→"Acq Time(ms)":u32, "Datas"=w658:i32[][][])  [unwired: 1 out]
            "Datas" <- w658
            n255 = for {
              tunnel: [w688] -> w671 mode=concatenating
              tunnel: [w687] -> w670 mode=concatenating
              tunnel: [w686] -> w669 mode=concatenating
              tunnel: [w685] -> w665 mode=concatenating
              tunnel: w659 -> [w684]
              tunnel: w658 -> [w683] mode=indexing
              n256 = for {
                tunnel: w683 -> [w695] mode=indexing
                tunnel: [w694] -> w687 mode=indexing
                tunnel: [w693] -> w686 mode=indexing
                n257 = Array Max & Min(array=w695) -> (max value=w693:i32, max index (indices)=w694:i32)  [unwired: 2 out]
              }
              n258 = case shown="Faux" w684 {
                tunnel: [w690 w692] -> w688
                tunnel: w683 -> [w689 w692]
                tunnel: [w689 w691] -> w685
                frame False {
                  n259 = Transpose 2D Array(2D array=w689) -> (transposed array=w690:i32[][])
                }
                frame True {
                  n260 = Transpose 2D Array(2D array=w692) -> (transposed array=w691:i32[][])
                }
              }
            }
            "Max Intensity" <- w669
            "Max X Position" <- w670
            n261 = call <userlib>:"Symphony ReadTemp.vi"("error in (no error)"=w674, "JYCCDLib.IJYCCDReqd"=w673) -> ("error out"=w657:errorcluster, "AcqTime"=w672:u32, "Current Temperature"=w663:dbl)  [unwired: 5 in, 1 out]
            n262 = local write "Current Temp"(w663) -> ()
            n263 = local write "T_AcqTime"(w672) -> ()
            n264 = local read "Continuous Acq."() -> (w677:bool)
            n265 = local write "Spectral Graph"(w665) -> ()
            n266 = local write "Image Graph"(w671) -> ()
            n267 = local read "RemCom"() -> (w661:bool)
            n268 = case shown="Faux" w677 {
              tunnel: w657 -> [w711 w712]
              tunnel: [w711 w714] -> w678
              tunnel: w676 -> [_ w713]
              frame False {
              }
              frame True {
                n269 = case shown="Pas d'erreur" w712 {
                  selector: w712 -> [w715 w720]
                  tunnel: [w717 w720] -> w714
                  tunnel: w713 -> [w716 _]
                  frame No Error {
                    n270 = Enqueue Element(queue=w716, element=cluster{"Message":string, "Data":variant, i32} {"Message"="AcqImage", "Data"=variant, 0} ("ClassQueue"), error in (no error)=w715) -> (error out=w717:errorcluster)  [unwired: 1 in, 2 out]
                  }
                  frame Error {
                    n271 = local write "Continuous Acq."(FALSE ("Continuous Acq.")) -> ()
                  }
                }
              }
            }
            n272 = case shown="Vrai" w661 {
              tunnel: w658 -> [_ w707]
              tunnel: w663 -> [_ w706]
              tunnel: w657 -> [w696 w705]
              tunnel: [w696 w700] -> w660
              tunnel: w662 -> [_ w703]
              tunnel: w659 -> [_ w697]
              frame False {
              }
              frame True {
                n273 = Bundle("Datas"=w707, "Current Temperature"=w706, "Image mode"=w697) -> (w708:T9)  [unwired: 1 in]
                n274 = Bundle By Name(cluster=T2 {"Message"="AcqDone", "Data"=variant, "Code"=0} ("ClassQueue"), "Data"=w708, "Code"=w703) -> (w704:T2)
                n275 = Bundle By Name(cluster=T2 {"Message"="CommandError", "Data"=variant, "Code"=0} ("ClassQueue"), "Code"=w703) -> (w701:T2)
                n276 = local read "ClientConn"() -> (w710:refnum<k13>)
                n277 = Select(t=w701, s=w705, f=w704) -> (s? t:f=w699:T2)
                n278 = local write "RemCom"(FALSE ("RemCom")) -> ()
                n279 = DataSocket Write(10:w699, 11:w710) -> (0:w700:errorcluster)  [unwired: 2 in, 2 out]
              }
            }
            n280 = Array Max & Min(array=w669) -> (max value=w668:i32, min value=w667:i32)  [unwired: 2 out]
            n281 = Subtract(x=w668, y=w667) -> (x-y=→"Delta":i32)
            n282 = Merge Errors(w660, w678) -> (w664:errorcluster)
          }
        }
      }
      n283 = while {
        tunnel: w13 -> [w20]
        shift-right: [w17] -> w11
        shift-left: w6 -> [w18]
        stop <- w19 stop-if-true
        n284 = event shown="[0] Timeout" {
          selector: _ -> [_ _ _ _ _ _ _ _ _ _ _ _]
          dyn-events: _ -> [_ _ _ _ _ _ _ _ _ _ _ _]
          timeout: 100 -> [_ _ _ _ _ _ _ _ _ _ _ _]
          tunnel: w20 -> [w22 w80 w96 w113 w120 w124 w130 w142 w152 w165 w177 w189]
          tunnel: [_ _ _ _ _ _ _ _ _ _ w174 w186] -> w19
          tunnel: w18 -> [w23 w79 w95 w112 w119 w123 w129 w141 w151 w164 w176 w188]
          tunnel: [w24 w78 w94 w111 w118 w122 w128 w140 w150 w163 w175 w187] -> w17
          event Timeout {
            n285 = event-data() -> ()  [unwired: 1 in, 2 out]
            n286 = case shown="Pas d'erreur" w23 {
              selector: w23 -> [w33 w75]
              tunnel: [w30 w76] -> w24
              tunnel: w22 -> [w32 _]
              frame No Error {
                n287 = case shown="Vrai" "Server Running" {
                  tunnel: w33 -> [w56 w65]
                  tunnel: [w56 w59] -> w28
                  tunnel: w32 -> [w55 w62]
                  tunnel: [w55 w58] -> w29
                  frame False {
                    # "server not operating"
                  }
                  frame True {
                    (unwired) 1 ("Code")
                    # "Check for client message"
                    n288 = local read "ServerConn"() -> (w66:refnum<k13>)
                    n289 = DataSocket Read(8:w65, 9:100 ("ms timeout (10000)"), 10:T2 {"Message"="", "Data"=variant, "Code"=0} ("SympClient"), 11:w66) -> (0:w60:errorcluster, 1:w61:bool, 2:w57:T2)  [unwired: 1 in, 4 out]
                    n290 = case shown="Vrai" w61 {
                      tunnel: w62 -> [w71 w73]
                      tunnel: w57 -> [w72 _]
                      tunnel: w60 -> [w70 w74]
                      tunnel: [w69 w74] -> w59
                      tunnel: [w68 w73] -> w58
                      frame False {
                        n291 = local write "RemCom"(TRUE ("RemCom")) -> ()
                        n292 = Enqueue Element(queue=w71, element=w72, error in (no error)=w70) -> (queue out=w68:refnum<queue>, error out=w69:errorcluster)  [unwired: 1 in, 1 out]
                      }
                      frame True {
                        # "no new \nmessage"
                      }
                    }
                  }
                }
                n293 = Unbundle By Name(w28) -> ("status"=w27:bool)
                n294 = And(x="Server Running", y=w27) -> (x .and. y?=w26:bool)
                n295 = case shown="Faux" "ReadTemp" {
                  tunnel: w28 -> [w35 w48]
                  tunnel: [w35 w47] -> w30
                  tunnel: w29 -> [_ w46]
                  frame False {
                  }
                  frame True {
                    n296 = local read "T_AcqTime"() -> (w45:u32)
                    n297 = Tick Count (ms)() -> (millisecond timer value=w44:u32)
                    n298 = local read "Aquiring"() -> (w41:bool)
                    n299 = local read "TempReq"() -> (w37:bool)
                    n300 = Subtract(x=w44, y=w45) -> (x-y=w43:u32)
                    n301 = Not(x=w41) -> (.not. x?=w40:bool)
                    n302 = Greater?(x=w43, y="T_Acq_Int") -> (0:w38:bool)
                    n303 = Not(x=w37) -> (.not. x?=w36:bool)
                    n304 = Compound Arithmetic op=AND(w36, w38, w40) -> (w39:bool)
                    n305 = case shown="Vrai" w39 {
                      selector: w39 -> [_ w50]
                      tunnel: w48 -> [w49 w53]
                      tunnel: [w49 w52] -> w47
                      tunnel: w46 -> [_ w51]
                      frame False {
                      }
                      frame True {
                        n306 = Enqueue Element(queue=w51, element=cluster{"Message":string, "Data":variant, i32} {"Message"="AcqTemp", "Data"=variant, 0} ("ClassQueue"), error in (no error)=w53) -> (error out=w52:errorcluster)  [unwired: 1 in, 2 out]
                        "TempReq" <- w50
                      }
                    }
                  }
                }
                n307 = case shown="Faux" w26 {
                  frame False {
                  }
                  frame True {
                    n308 = local write "Server Running"(FALSE ("Launch server")) -> ()
                  }
                }
              }
              frame Error {
                n309 = call <vilib>:"Simple Error Handler.vi"("error in (no error)"=w75) -> ("error out"=w77:errorcluster)  [unwired: 4 in, 4 out]
                n310 = call <vilib>:"Clear Errors.vi"("error in (no error)"=w77) -> ("error out"=w76:errorcluster)  [unwired: 5 in, 1 out]
              }
            }
          }
          event "Y Bins": Key Down {
            n311 = event-data() -> ("Char"=w82:i16)  [unwired: 1 in]
            n312 = Equal To 0?(x=w82) -> (x = 0?=w81:bool)
            n313 = case shown="Vrai" w81 {
              tunnel: w80 -> [_ w87]
              tunnel: w79 -> [w83 w85]
              tunnel: [w83 w86] -> w78
              frame False {
              }
              frame True {
                n314 = Wait (ms)(milliseconds to wait=u32 200) -> (millisecond timer value=w84:u32)
                n315 = flat-sequence {
                  tunnel: w87 -> [w91]
                  tunnel: [w90] -> w86
                  tunnel: w85 -> [w89]
                  tunnel: w84 -> [_]
                  frame #0 {
                    n316 = Enqueue Element(queue=w91, element=cluster{"Message":string, "Data":variant, i32} {"Message"="SetArea", "Data"=variant, 0} ("ClassQueue"), error in (no error)=w89) -> (error out=w90:errorcluster)  [unwired: 1 in, 2 out]
                  }
                }
              }
            }
          }
          event "SetArea": Value Change {
            n317 = event-data() -> ("NewVal"=w93:bool)  [unwired: 1 in]
            n318 = case shown="Vrai" w93 {
              tunnel: w96 -> [_ w102]
              tunnel: w95 -> [w97 w100]
              tunnel: [w97 w101] -> w94
              frame False {
              }
              frame True {
                n319 = Wait (ms)(milliseconds to wait=u32 200) -> (millisecond timer value=w99:u32)
                n320 = flat-sequence {
                  tunnel: w102 -> [w107]
                  tunnel: [w106] -> w101
                  tunnel: w100 -> [w105]
                  tunnel: w99 -> [_]
                  tunnel: [FALSE ("SetArea")] -> w98
                  frame #0 {
                    n321 = Enqueue Element(queue=w107, element=cluster{"Message":string, "Data":variant, i32} {"Message"="SetArea", "Data"=variant, 0} ("ClassQueue"), error in (no error)=w105) -> (error out=w106:errorcluster)  [unwired: 1 in, 2 out]
                  }
                }
                n322 = local write "SetArea"(w98) -> ()
              }
            }
          }
          event "Image mode": Value Change {
            n323 = event-data() -> ()  [unwired: 1 in, 1 out]
            n324 = Wait (ms)(milliseconds to wait=u32 200) -> (millisecond timer value=w109:u32)
            n325 = flat-sequence {
              tunnel: w113 -> [w116]
              tunnel: [w115] -> w111
              tunnel: w112 -> [w114]
              tunnel: w109 -> [_]
              frame #0 {
                n326 = Enqueue Element(queue=w116, element=cluster{"Message":string, "Data":variant, i32} {"Message"="SetArea", "Data"=variant, 0} ("ClassQueue"), error in (no error)=w114) -> (error out=w115:errorcluster)  [unwired: 1 in, 2 out]
              }
            }
          }
          event "Gain": Value Change {
            n327 = event-data() -> ()  [unwired: 1 in, 1 out]
            n328 = Enqueue Element(queue=w120, element=cluster{"Message":string, "Data":variant, i32} {"Message"="SetGain", "Data"=variant, 0} ("ClassQueue"), error in (no error)=w119) -> (error out=w118:errorcluster)  [unwired: 1 in, 2 out]
          }
          event "ADC": Value Change {
            n329 = event-data() -> ()  [unwired: 1 in, 1 out]
            n330 = Enqueue Element(queue=w124, element=cluster{"Message":string, "Data":variant, i32} {"Message"="SetADC", "Data"=variant, 0} ("ClassQueue"), error in (no error)=w123) -> (error out=w122:errorcluster)  [unwired: 1 in, 2 out]
          }
          event "AcquireImage": Value Change {
            n331 = event-data() -> ("NewVal"=w127:bool)  [unwired: 1 in]
            n332 = case shown="Vrai" w127 {
              tunnel: w130 -> [_ w137]
              tunnel: w129 -> [w132 w136]
              tunnel: [w132 w135] -> w128
              tunnel: [FALSE FALSE] -> w126
              frame False {
              }
              frame True {
                n333 = Enqueue Element(queue=w137, element=cluster{"Message":string, "Data":variant, i32} {"Message"="AcqImage", "Data"=variant, 0} ("ClassQueue"), error in (no error)=w136) -> (error out=w135:errorcluster)  [unwired: 1 in, 2 out]
                n334 = Wait (ms)(milliseconds to wait=u32 200) -> ()  [unwired: 1 out]
              }
            }
            n335 = local write "AcquireImage"(w126) -> ()
          }
          event "Continuous Acq.": Value Change {
            n336 = event-data() -> ("NewVal"=w139:bool)  [unwired: 1 in]
            n337 = case shown="Vrai" w139 {
              tunnel: w142 -> [_ w146]
              tunnel: w141 -> [w143 w145]
              tunnel: [w143 w144] -> w140
              frame False {
              }
              frame True {
                n338 = Enqueue Element(queue=w146, element=cluster{"Message":string, "Data":variant, i32} {"Message"="AcqImage", "Data"=variant, 0} ("ClassQueue"), error in (no error)=w145) -> (error out=w144:errorcluster)  [unwired: 1 in, 2 out]
              }
            }
          }
          event "Int_time(ms)": Key Down {
            n339 = event-data() -> ("Char"=w149:i16)  [unwired: 1 in]
            n340 = Equal To 0?(x=w149) -> (x = 0?=w148:bool)
            n341 = case shown="Vrai" w148 {
              tunnel: w152 -> [_ w158]
              tunnel: w151 -> [w153 w157]
              tunnel: [w153 w156] -> w150
              frame False {
              }
              frame True {
                n342 = Wait (ms)(milliseconds to wait=u32 200) -> (millisecond timer value=w155:u32)
                n343 = flat-sequence {
                  tunnel: w158 -> [w161]
                  tunnel: w157 -> [w160]
                  tunnel: [w159] -> w156
                  tunnel: w155 -> [_]
                  frame #0 {
                    n344 = Enqueue Element(queue=w161, element=cluster{"Message":string, "Data":variant, i32} {"Message"="SetInteg", "Data"=variant, 0} ("ClassQueue"), error in (no error)=w160) -> (error out=w159:errorcluster)  [unwired: 1 in, 2 out]
                  }
                }
              }
            }
          }
          event "Init": Value Change {
            n345 = event-data() -> ("NewVal"=w166:bool)  [unwired: 1 in]
            n346 = case shown="Vrai" w166 {
              tunnel: w165 -> [_ w168]
              tunnel: w164 -> [w167 w169]
              tunnel: [w167 w170] -> w163
              frame False {
              }
              frame True {
                n347 = Enqueue Element(queue=w168, element=T2 {"Message"="InitCam", "Data"=variant, "Code"=0}, error in (no error)=w169) -> (error out=w170:errorcluster)  [unwired: 1 in, 2 out]
                n348 = local write "Init"(FALSE ("Init")) -> ()
              }
            }
          }
          event Panel Close? {
            n349 = event-data() -> ()  [unwired: 1 in, 4 out]
            n350 = Two Button Dialog(message="Quit Program?") -> (T button?=w174:bool)  [unwired: 2 in]
            n351 = case shown="Vrai" w174 {
              tunnel: w177 -> [_ w184]
              tunnel: w176 -> [w180 w183]
              tunnel: [w180 w182] -> w175
              tunnel: [TRUE FALSE ("Stop")] -> w173
              frame False {
              }
              frame True {
                n352 = Enqueue Element(queue=w184, element=cluster{"Message":string, "Data":variant, i32} {"Message"="Stop", "Data"=variant, 0}, error in (no error)=w183) -> (error out=w182:errorcluster)  [unwired: 1 in, 2 out]
              }
            }
            n353 = event-data("Discard?"=w173) -> ()  [unwired: 1 in, 1 out]
          }
          event "Stop": Value Change {
            n354 = event-data() -> ()  [unwired: 1 in, 6 out]
            n355 = Two Button Dialog(message="Quit Program?") -> (T button?=w186:bool)  [unwired: 2 in]
            n356 = case shown="Vrai" w186 {
              tunnel: w189 -> [_ w195]
              tunnel: w188 -> [w191 w194]
              tunnel: [w191 w192] -> w187
              frame False {
              }
              frame True {
                n357 = local write "Stop"(FALSE ("Stop")) -> ()
                n358 = Enqueue Element(queue=w195, element=cluster{"Message":string, "Data":variant, i32} {"Message"="Stop", "Data"=variant, 0}, error in (no error)=w194) -> (error out=w192:errorcluster)  [unwired: 1 in, 2 out]
              }
            }
          }
        }
      }
      n359 = Close Reference(reference=w7, error in (no error)=w8) -> (error out=w9:errorcluster)
      n360 = Merge Errors(w9, w11) -> (w14:errorcluster)
    }
    frame Error {
    }
  }
  "error out" <- w1
